vi "ShootTask.vi"() -> (0 "DoneReloading":bool)   [LabVIEW 2015]
uses:
  <vilib>/Rock Robotics/WPI/Solenoid/WPI_SolenoidValue.ctl
  GeneralGlobals.vi
  VisionGlobals.vi
  MotorPositionGlobals.vi
  <vilib>/Rock Robotics/WPI/Solenoid/WPI_SolenoidSetEnum.vi
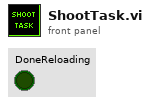
[diagram p1: front panel]
types:
  T1 = typedef "WPI_SolenoidValue.ctl" = enum16{"Off", "On", "Forward", "Reverse"}
  T2 = typedef "WPI_SolenoidDevRef.ctl" = cluster{"DevStatus":errorcluster, "Pneumatics Control Module":u8, "Forward Solenoid Channel":T3, "Reverse Solenoid Channel":T3}
  T3 = typedef "WPI_SolenoidChannel.ctl" = enum8{"Solenoid 0", "Solenoid 1", "Solenoid 2", "Solenoid 3", "Solenoid 4", "Solenoid 5", "Solenoid 6", "Solenoid 7", "Invalid"}
  T4 = typedef "WPI_MotorControlDeviceRef.ctl" = cluster{"DeviceStatus":errorcluster, "Type":T5, "PWM":cluster{"PWM Channel":T6, "DeadBand":T7}, "CAN":cluster{"Device Number":u8, "Control Mode":T8, "Semaphore":T9, "Max Vout":dbl, "TalonSRX Control Mode":T10}, "Invert":bool}
  T5 = typedef "WPI_MotorControlType.ctl" = enum16{"PWM", "CAN", "CANTalonSRX"}
  T6 = typedef "FPGA_DIOPWMChannel.ctl" = enum8{"PWM 0", "PWM 1", "PWM 2", "PWM 3", "PWM 4", "PWM 5", "PWM 6", "PWM 7", "PWM 8", "PWM 9", "PWM MXP 0", "PWM MXP 1", "PWM MXP 2", "PWM MXP 3", "PWM MXP 4", "PWM MXP 5", "PWM MXP 6", "PWM MXP 7", "PWM MXP 8", "PWM MXP 9", "Invalid"}
  T7 = typedef "WPI_PWMDeadband.ctl" = cluster{"Name":string, "maxPositivePwm":i32, "minPositivePwm":i32, "centerPwm":i32, "maxNegativePwm":i32, "minNegativePwm":i32, "angularRange":u16}
  T8 = typedef "WPI_CANJaguar_ControlMode.ctl" = enum8{"Percent VBus", "Current", "Speed", "Position", "Voltage"}
  T9 = typedef "Semaphore RefNum" = refnum<k1>
  T10 = typedef "WPI_CANTalonSRX_APIControlMode.ctl" = enum8{"Percent VBus", "Speed", "Position", "Slave", "Unchanged / Invalid", "Voltage Compensation", "Current", "Motion Profile"}
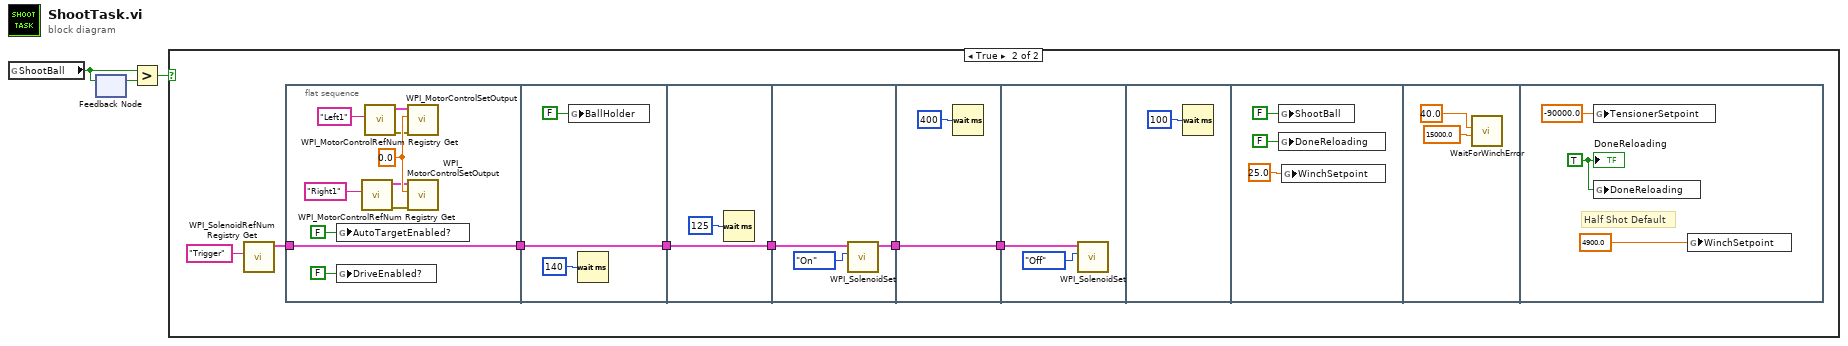
[diagram p0: block diagram]
diagram:
  n1 = global read "GeneralGlobals.vi" "ShootBall"() -> (w3:bool)
  n2 = feedback-in #1(w3) -> ()
  n3 = feedback #1() -> (w2:bool)  [unwired: 1 in]
  n4 = Greater?(x=w3, y=w2) -> (0:w1:bool)
  n5 = case shown="True" w1 {
    frame False {
    }
    frame True {
      n6 = call <vilib>:"WPI_SolenoidRefNum Registry Get.vi"("refnum name"="Trigger") -> ("SolenoidDevRef"=w5:T2)  [unwired: 9 in, 1 out]
      n7 = flat-sequence {
        tunnel: [w20] -> w10
        tunnel: w5 -> [w20]
        tunnel: w10 -> [w23]
        tunnel: [w23] -> w9
        tunnel: w9 -> [w25]
        tunnel: [w25] -> w8
        tunnel: [w26] -> w7
        tunnel: w8 -> [w27]
        tunnel: w7 -> [w29]
        tunnel: [w29] -> w6
        tunnel: w6 -> [w31]
        frame #0 {
          w16 = 0.0
          n8 = global write "VisionGlobals.vi" "AutoTargetEnabled?"(FALSE ("AutoTargetEnabled?")) -> ()
          n9 = global write "VisionGlobals.vi" "DriveEnabled?"(FALSE ("DriveEnabled?")) -> ()
          n10 = call <vilib>:"WPI_MotorControlRefNum Registry Get.vi"("refnum name"="Right1") -> ("error out"=w14:errorcluster, "MotorControlDevRef"=w15:T4)  [unwired: 9 in]
          n11 = call <vilib>:"WPI_MotorControlRefNum Registry Get.vi"("refnum name"="Left1") -> ("error out"=w12:errorcluster, "MotorControlDevRef"=w13:T4)  [unwired: 9 in]
          n12 = call <vilib>:"WPI_MotorControlSetOutput.vi"("error in (no error)"=w12, "Output"=w16, "MotorControlDevRef"=w13) -> ()  [unwired: 6 in, 3 out]
          n13 = call <vilib>:"WPI_MotorControlSetOutput.vi"("error in (no error)"=w14, "Output"=w16, "MotorControlDevRef"=w15) -> ()  [unwired: 6 in, 3 out]
        }
        frame #1 {
          n14 = global write "MotorPositionGlobals.vi" "BallHolder"(FALSE ("BallHolder")) -> ()
          n15 = Wait (ms)(milliseconds to wait=u32 140) -> ()  [unwired: 1 out]
        }
        frame #2 {
          n16 = Wait (ms)(milliseconds to wait=u32 125) -> ()  [unwired: 1 out]
        }
        frame #3 {
          n17 = call-poly <vilib>:"WPI_SolenoidSet.vi"("Value"=WPI_SolenoidValue."On", "SolenoidDevRef"=w27) -> ("SolenoidDevRef"=w26:T2)  [unwired: 8 in, 1 out]
        }
        frame #4 {
          n18 = Wait (ms)(milliseconds to wait=u32 400) -> ()  [unwired: 1 out]
        }
        frame #5 {
          n19 = call-poly <vilib>:"WPI_SolenoidSet.vi"("Value"=WPI_SolenoidValue."Off", "SolenoidDevRef"=w31) -> ()  [unwired: 8 in, 2 out]
        }
        frame #6 {
          n20 = Wait (ms)(milliseconds to wait=u32 100) -> ()  [unwired: 1 out]
        }
        frame #7 {
          n21 = global write "GeneralGlobals.vi" "ShootBall"(FALSE ("ShootBall")) -> ()
          n22 = global write "GeneralGlobals.vi" "DoneReloading"(FALSE ("ShootBall")) -> ()
          n23 = global write "MotorPositionGlobals.vi" "WinchSetpoint"(25.0 ("WinchPosition")) -> ()
        }
        frame #8 {
          n24 = call "WaitForWinchError.vi"("Timeout (ms)"=15000.0, "AllowedError"=40.0) -> ()  [unwired: 9 in, 1 out]
        }
        frame #9 {
          w39 = TRUE ("ShootBall")
          # "Half Shot Default"
          n25 = global write "MotorPositionGlobals.vi" "TensionerSetpoint"(-90000.0 ("TensionerSetpoint")) -> ()
          n26 = global write "GeneralGlobals.vi" "DoneReloading"(w39) -> ()
          n27 = global write "MotorPositionGlobals.vi" "WinchSetpoint"(4900.0 ("WinchPosition")) -> ()
          "DoneReloading" <- w39
        }
      }
    }
  }
